vi "Write VISA resource name.vi"(10 "VISA resource name":refnum<visa-resource-name>, 11 "Instrumento in":refnum<class "Instrumento.lvclass">) -> (3 "Instrumento out":refnum<class "Instrumento.lvclass">)   [LabVIEW 2020, in "Instrumento.lvclass"]
uses:
  Instrumento.lvclass
  Instrumento.lvclass/Instrumento.ctl
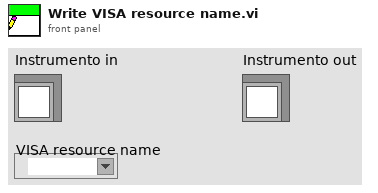
[diagram p1: front panel]
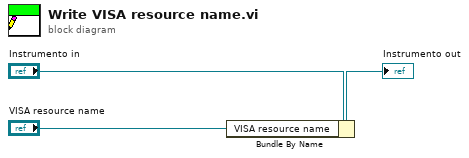
[diagram p0: block diagram]
diagram:
  n1 = Bundle By Name(cluster="Instrumento in", "VISA resource name"="VISA resource name") -> (→"Instrumento out":refnum<class "Instrumento.lvclass">)
